vi "HovaCAL TestRun Values.vi"() -> (1 "Cluster.PumpModeGeneral-Cluster":T2, 2 "MFC Output":T4 {"Actual Flow" format="%.2f"}, 3 "Cluster.Temp Cluster":T3(array[cluster]), 4 "Water-Cluster out":cluster{"water conc SP":dbl, "water conc":dbl}, 5 "MFC Output Array":T1[](array[typedef]) {"Input Concentration" format="%.2f"; "Output Setpoint" format="%.2f"; "flow expected" format="%.2f"; "flow actual" format="%.2f"; "output concentration dry" format="%.2f"; "output concentration" format="%.2f"})   [LabVIEW 2020, in "EPA 1065.lvlib" / "HovaCAL Interference verificaton.lvlib"]
uses:
  HovaCAL Interference verificaton.lvlib
  Linearisierung V2/Gasteiler/HovaCAL_Interface/Controls/Flow Anzeige.ctl
  Linearisierung V2/Gasteiler/HovaCAL_Interface/Controls/Pumpe Status Anzeige.ctl
  Aktion FGV Interference.ctl
  Linearisierung V2/Gasteiler/HovaCAL_Interface/Kommunikation/Aktion_FGV_HovaCAL_Interface_SetData.ctl
  Linearisierung V2/Gasteiler/HovaCAL_Interface/Controls/Controls.lvlib
  Linearisierung V2/Gasteiler/HovaCAL_Interface/Kommunikation/Kommunikation.lvlib
  Linearisierung V2/Gasteiler/HovaCAL_Interface/Controls/MFC Output plus Input Output Concentrations.ctl
panel:
  # "l/min"
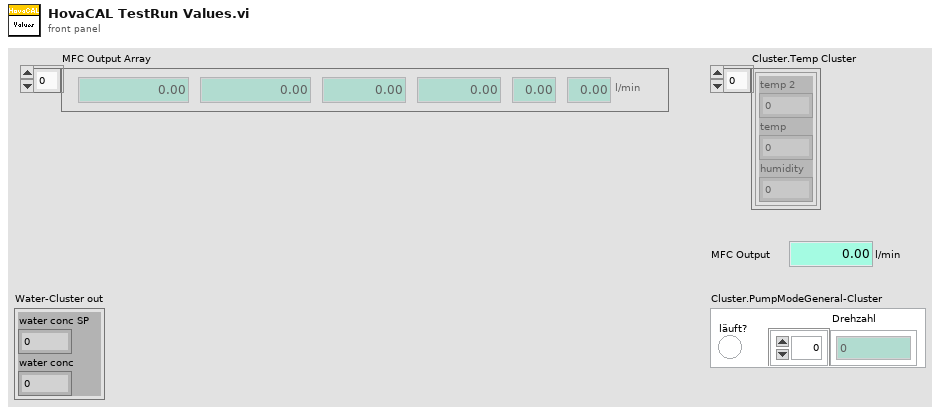
[diagram p1: front panel]
types:
  T1 = typedef "Linearisierung v2.lvlib/Gasteiler.lvlib/HovaCAL_Interface.lvlib/Controls.lvlib/MFC Output plus Input Output Concentrations.ctl" = cluster{"Input Concentration":dbl, "Output Setpoint":dbl, "output concentration":dbl, "output concentration dry":dbl, "flow actual":dbl, "flow expected":dbl}
  T2 = typedef "Linearisierung v2.lvlib/Gasteiler.lvlib/HovaCAL_Interface.lvlib/Controls.lvlib/Pumpe Status Anzeige.ctl" = cluster{"running?":bool, "Speed":dbl[]}
  T3 = cluster{"temp 2":dbl, "temp":dbl, "humidity":dbl}[]
  T4 = typedef "Linearisierung v2.lvlib/Gasteiler.lvlib/HovaCAL_Interface.lvlib/Controls.lvlib/Flow Anzeige.ctl" = cluster{"Actual Flow":dbl}
  T5 = typedef "EPA 1065.lvlib/HovaCAL Interference verificaton.lvlib/Aktion FGV Interference.ctl" = enum16{"Lesen", "TestKonfig", "TestSetting", "Einheiten", "Ergebnis", "Laden", "Tabelle", "Speichern", "löschen"}
  T6 = typedef "Linearisierung v2.lvlib/Gasteiler.lvlib/HovaCAL_Interface.lvlib/Kommunikation.lvlib/Aktion_FGV_HovaCAL_Interface_SetData.ctl" = enum16{"lesen", "Konzentrationen", "Pumpen Parameter", "Pumpe Konzentration", "Pumpe run", "Temperaturen", "Fluss", "Limits", "init"}
  T7 = cluster{"temp 2":dbl, "temp":dbl, "humidity":dbl}
  T8 = cluster{"input concentration setpoint":dbl, "output concentration setpoint":dbl}[]
  T9 = typedef "Linearisierung v2.lvlib/Gasteiler.lvlib/HovaCAL_Interface.lvlib/Controls.lvlib/Pump Concentration.ctl" = cluster{"reagent conc SP":dbl, "water conc SP":dbl}
  T10 = cluster{"water conc SP":dbl, "water conc SP":dbl}
  T11 = cluster{"temp SP":dbl, "temp":dbl, "humidity":dbl}[]
  T12 = typedef "EPA 1065.lvlib/HovaCAL Interference verificaton.lvlib/TestKonfig.ctl" = cluster{"TestKonfig H2O":T13, "TestKonfig Interferent":T19}
  T13 = typedef "EPA 1065.lvlib/HovaCAL Interference verificaton.lvlib/TestKonfig H2O.ctl" = cluster{"Modus":T14, "Komponente:":u16, "Eingangs Konzentration:":dbl, "Einheit":T15, "Anzahl Stufen":sgl, "Zeitdauer Stufen":sgl, "Max Fehler":sgl, "zusätzliche Zeitdauer Erster Punkt":sgl, "Punkte umkehren":bool, "Stufen Tabelle":T16, "HovaCAL Flow Input Cluster":T17, "HovaCAL Temperature":T18}
  T14 = typedef "EPA 1065.lvlib/HovaCAL Interference verificaton.lvlib/Modus.ctl" = u16
  T15 = typedef "Linearisierung v2.lvlib/SpanEinstellungen.lvlib/Einheit.ctl" = enum16{"ppm", "%"}
  T16 = typedef "Linearisierung v2.lvlib/Gasteiler.lvlib/Stufen Tabelle 10 Stufen.ctl" = string[][]
  T17 = typedef "Linearisierung v2.lvlib/Gasteiler.lvlib/HovaCAL_Interface.lvlib/Controls.lvlib/Flow Einstellung.ctl" = cluster{"HovaCAL Flow Input Cluster":dbl}
  T18 = typedef "Linearisierung v2.lvlib/Gasteiler.lvlib/HovaCAL_Interface.lvlib/Controls.lvlib/Temp Sollwerte Anzeige.ctl" = dbl[]
  T19 = typedef "EPA 1065.lvlib/HovaCAL Interference verificaton.lvlib/TestKonfig Interferents.ctl" = cluster{"MFC1":enum16{"MFC 1"}, "Eingangs Konzentration MFC1":dbl, "Einheit MFC1 Eingang":T15, "Ausgangs Konzentration MFC1":dbl, "Einheit MFC1 Ausgang":T15, "MFC2":T20, "Referenz-Interferent:":u16, "Gasflaschen Nr MFC2":string, "Accuracy MFC2":string, "Eingangs Konzentration MFC2":dbl, "Einheit MFC2 Eingang":T15, "Ausgangs Konzentration MFC2":dbl, "Einheit MFC2 Ausgang":T15, "MFC3":T20, "Kontroll-Interferent:":u16, "Gasflaschen Nr MFC3":string, "Accuracy MFC3":string, "Eingangs Konzentration MFC3":dbl, "Einheit MFC3 Eingang":T15, "Ausgangs Konzentration MFC3":dbl, "Einheit MFC3 Ausgang":T15, "Gasflasche MFC2":T21, "Gasflasche MFC3":T21}
  T20 = typedef "EPA 1065.lvlib/HovaCAL Interference verificaton.lvlib/MFCAuswahl.ctl" = u16
  T21 = typedef "System Einstellungen V2.lvlib/Gasflasche Auswahl.ctl" = u16
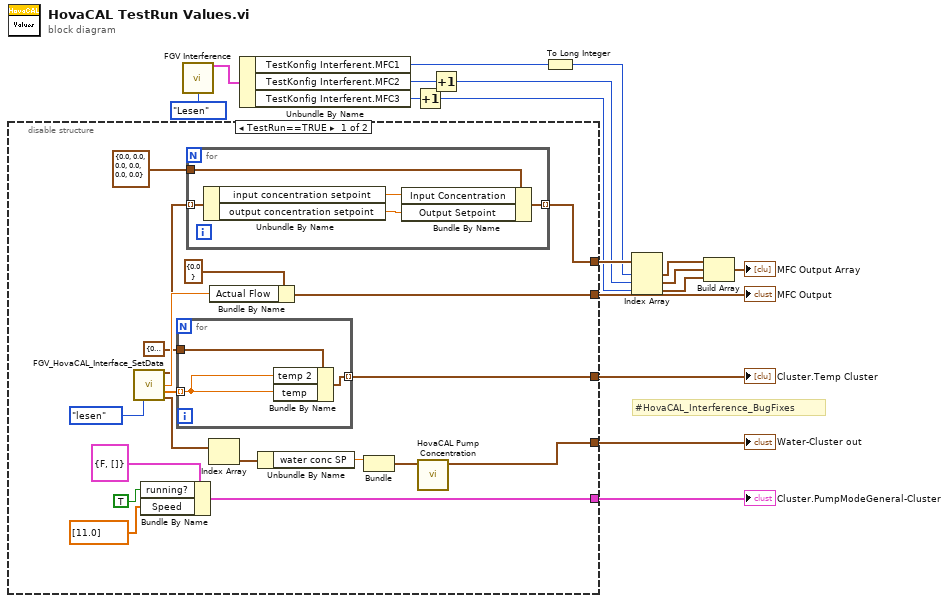
[diagram p0: block diagram]
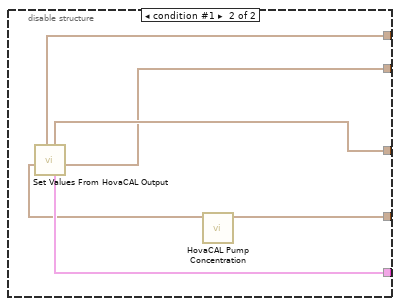
[diagram p2: hidden frame]
diagram:
  # "#HovaCAL_Interference_BugFixes"
  n1 = disable-structure shown="TestRun==TRUE" {
    disable-tunnel: [w33 w49] -> w17
    disable-tunnel: [w31 w50] -> w16
    disable-tunnel: [w27 w48] -> w15
    disable-tunnel: [w18 w45] -> w14
    disable-tunnel: [w21 w46] -> w2
    frame condition #0 (active) {
      n2 = call "FGV_HovaCAL_Interface_SetData.vi"("Aktion"=Aktion_FGV_HovaCAL_Interface_SetData."lesen") -> ("Set Values Cluster out"=w20:T8, "total flow setpoint out"=w35:dbl, "Temperature out"=w36:dbl[], "Pump Concentrations-Cluster out"=w25:T9[])  [unwired: 8 in, 3 out]
      n3 = Bundle By Name(cluster=T2 {"running?"=FALSE, "Speed"=[]} ("Cluster.PumpModeGeneral-Cluster"), "running?"=TRUE, "Speed"=dbl[] [11.0]) -> (w27:T2)
      n4 = for {
        tunnel: T7 {"temp 2"=0.0, "temp"=0.0, "humidity"=0.0} ("Temp Cluster") -> [w44]
        tunnel: [w43] -> w31 mode=indexing
        tunnel: w36 -> [w42] mode=indexing
        n5 = Bundle By Name(cluster=w44, "temp 2"=w42, "temp"=w42) -> (w43:T7)
      }
      n6 = for {
        tunnel: w20 -> [w41] mode=indexing
        tunnel: T1 {"Input Concentration"=0.0, "Output Setpoint"=0.0, "output concentration"=0.0, "output concentration dry"=0.0, "flow actual"=0.0, "flow expected"=0.0} ("Actual Values Cluster") -> [w40]
        tunnel: [w37] -> w18 mode=indexing
        n7 = Unbundle By Name(w41) -> ("input concentration setpoint"=w39:dbl, "output concentration setpoint"=w38:dbl)
        n8 = Bundle By Name(cluster=w40, "Input Concentration"=w39, "Output Setpoint"=w38) -> (w37:T1)
      }
      n9 = Index Array(array=w25) -> (element=w24:T9)  [unwired: 1 in]
      n10 = Bundle By Name(cluster=T4 {"Actual Flow"=0.0} ("MFC Output"), "Actual Flow"=w35) -> (w33:T4)
      n11 = Unbundle By Name(w24) -> ("water conc SP"=w23:dbl)
      n12 = Bundle("water conc SP"=w23, "water conc SP"=w23) -> (w22:T10)  [unwired: 1 in]
      n13 = call "HovaCAL Pump Concentration.vi"("Water-Cluster out (Eingang)"=w22) -> ("Water-Cluster out (Ausgang)"=w21:cluster{"water conc SP":dbl, "water conc":dbl})  [unwired: 10 in]
    }
    frame condition #1 {
      n14 = call "Set Values From HovaCAL Output.vi"() -> ("Cluster.Flow Output Cluster (Ausgang)"=w49:cluster{"total flow":dbl}, "Cluster.PumpModeGeneral-Cluster"=w48:cluster{"running?":bool, "Speed":dbl[]}, "Cluster.Temp Cluster"=w50:T11, "MFC Input/Output Concentrations (Ausgang)"=w45:T1[], "Water-Cluster out"=w47:cluster{"water conc SP":dbl, "water conc":dbl})  [unwired: 1 in, 6 out]
      n15 = call "HovaCAL Pump Concentration.vi"("Water-Cluster out (Eingang)"=w47) -> ("Water-Cluster out (Ausgang)"=w46:cluster{"water conc SP":dbl, "water conc":dbl})  [unwired: 10 in]
    }
  }
  "MFC Output" <- w17
  "Cluster.Temp Cluster" <- w16
  "Cluster.PumpModeGeneral-Cluster" <- w15
  "Water-Cluster out" <- w2
  n16 = call "FGV Interference.vi"("Aktion FGV Interference"=Aktion_FGV_Interference."Lesen") -> ("TestKonfig"=w12:T12)  [unwired: 9 in, 5 out]
  n17 = Unbundle By Name(w12) -> ("TestKonfig Interferent.MFC1"=w11:enum16{"MFC 1"}, "TestKonfig Interferent.MFC2"=w10:T20, "TestKonfig Interferent.MFC3"=w9:T20)
  n18 = Increment(x=w9) -> (x+1=w4:T20)
  n19 = Increment(x=w10) -> (x+1=w5:T20)
  n20 = To Long Integer(number=w11) -> (32bit integer=w3:i32)
  n21 = Index Array(array=w14, index #1=w3, index #2=w5, index #3=w4) -> (element #1=w8:T1, element #2=w7:T1, element #3=w6:T1)
  n22 = Build Array(w8, w7, w6) -> (→"MFC Output Array":T1[])
